vi "FRCts20_EspEngine_SearchBrowser.vi"(8 "error in (no error)":errorcluster, 10 "SearchBrowser":T1, 11 "httpRequestID":u32) -> (0 "error out":errorcluster, 3 "httpRequestID out":u32)   [LabVIEW 2014, in "FRCts20_EspEngine.lvlib"]
uses:
  FRCts20_EspEngine.lvlib
  TypeDefs/FRCts20_EspEngine_SearchBrowser.ctl
  <vilib>/wsapi/subVIs/Set String ESP Variable.vi
  <vilib>/wsapi/subVIs/Set Integer ESP Variable.vi
  FRCts20_EspEngine_FormatArrayOfKeysStrings.vi
  <vilib>/wsapi/NI_WebServices.lvlib
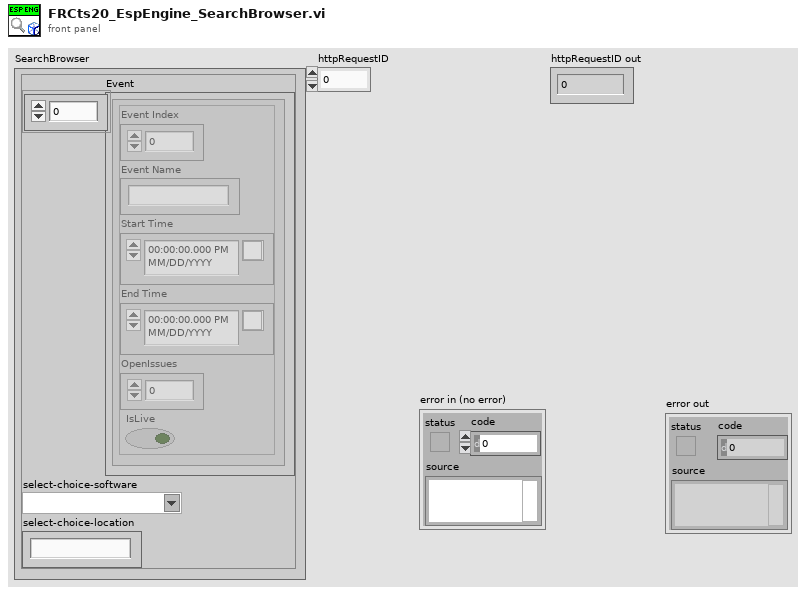
[diagram p1: front panel]
types:
  T1 = typedef "FRCts20_EspEngine.lvlib/FRCts20_EspEngine_SearchBrowser.ctl" = cluster{"Event":cluster{"Event Index":u32, "Event Name":string, "Start Time":timestamp, "End Time":timestamp, "OpenIssues":u8, "IsLive":bool}[], "select-choice-software":string, "select-choice-location":string}
  T2 = cluster{"Event Index":u32, "Event Name":string, "Start Time":timestamp, "End Time":timestamp, "OpenIssues":u8, "IsLive":bool}[]
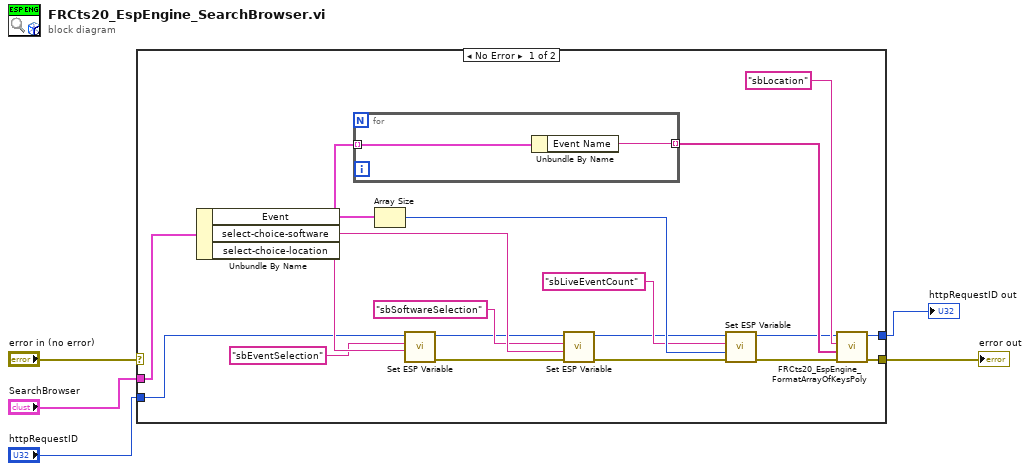
[diagram p0: block diagram]
diagram:
  n1 = case shown="No Error" "error in (no error)" {
    selector: "error in (no error)" -> [_ w27]
    tunnel: [w6 w27] -> w5
    tunnel: "SearchBrowser" -> [w24 _]
    tunnel: "httpRequestID" -> [w11 _]
    tunnel: [w7 _] -> w1
    frame No Error {
      n2 = Unbundle By Name(w24) -> ("Event"=w23:T2, "select-choice-software"=w17:string, "select-choice-location"=w16:string)
      n3 = for {
        tunnel: w23 -> [w26] mode=indexing
        tunnel: [w25] -> w20 mode=indexing
        n4 = Unbundle By Name(w26) -> ("Event Name"=w25:string)
      }
      n5 = Array Size(array=w23) -> (size(s)=w22:i32)
      n6 = call-poly <vilib>:"Set ESP Variable.vi"("value"=w16, "key"="sbEventSelection", "httpRequestID"=w11) -> ("error out"=w15:errorcluster, "httpRequestID out"=w10:u32)  [unwired: 7 in]
      n7 = call-poly <vilib>:"Set ESP Variable.vi"("error in (no error)"=w15, "value"=w17, "key"="sbSoftwareSelection", "httpRequestID"=w10) -> ("error out"=w14:errorcluster, "httpRequestID out"=w9:u32)  [unwired: 6 in]
      n8 = call-poly <vilib>:"Set ESP Variable.vi"("error in (no error)"=w14, "value"=w22, "key"="sbLiveEventCount", "httpRequestID"=w9) -> ("error out"=w18:errorcluster, "httpRequestID out"=w8:u32)  [unwired: 6 in]
      n9 = call-poly "FRCts20_EspEngine_FormatArrayOfKeysPoly.vi"("error IO"=w18, "Values"=w20, "KeyBaseName"="sbLocation", "httpRequestID"=w8) -> ("error IO"=w6:errorcluster, "httpRequestID out"=w7:u32)  [unwired: 6 in]
    }
    frame Error {
    }
  }
  "error out" <- w5
  "httpRequestID out" <- w1
